vi "Station_2_Home_Data.vi"(8 "Loader Home Data IN":T1={"Approach Velocity\n(In/Sec)"=1.0, "Creep Velocity\n(In/Sec)"=0.5, "Offset (In)"=0.0625, "OffsetVelocity\n(In/Sec)"=0.5, "AccDec\n(In/Sec/Sec)"=1.0, "Position (In)"=0.0} {"Position (In)" min=0.0 max=1.0 format="%.3f"; "AccDec\n(In/Sec/Sec)" min=0.01 max=20.0 format="%.2f"; "OffsetVelocity\n(In/Sec)" min=0.01 max=2.0 format="%.2f"; "Offset (In)" min=-1.0 max=1.0 format="%.3f"; "Creep Velocity\n(In/Sec)" min=0.5 max=1.0 format="%.2f"; "Approach Velocity\n(In/Sec)" min=0.01 max=2.0 format="%.2f"}, 9 "Z Home Data IN":T1={"Approach Velocity\n(In/Sec)"=1.0, "Creep Velocity\n(In/Sec)"=0.5, "Offset (In)"=-0.0625, "OffsetVelocity\n(In/Sec)"=0.5, "AccDec\n(In/Sec/Sec)"=1.0, "Position (In)"=5.75} {"Position (In)" format="%.3f"; "AccDec\n(In/Sec/Sec)" min=0.01 max=20.0 format="%.2f"; "OffsetVelocity\n(In/Sec)" min=0.01 max=2.0 format="%.2f"; "Offset (In)" min=-1.0 format="%.3f"; "Creep Velocity\n(In/Sec)" min=0.5 max=1.0 format="%.2f"; "Approach Velocity\n(In/Sec)" min=0.01 max=2.0 format="%.2f"}, 10 "Y Home Data IN":T1={"Approach Velocity\n(In/Sec)"=1.0, "Creep Velocity\n(In/Sec)"=0.5, "Offset (In)"=-0.0625, "OffsetVelocity\n(In/Sec)"=0.5, "AccDec\n(In/Sec/Sec)"=1.0, "Position (In)"=5.9} {"Position (In)" format="%.3f"; "AccDec\n(In/Sec/Sec)" min=0.01 max=20.0 format="%.2f"; "OffsetVelocity\n(In/Sec)" min=0.01 max=2.0 format="%.2f"; "Offset (In)" min=-1.0 max=1.0 format="%.3f"; "Creep Velocity\n(In/Sec)" min=0.5 max=1.0 format="%.2f"; "Approach Velocity\n(In/Sec)" min=0.01 max=2.0 format="%.2f"}, 11 "X Home Data IN":T2={"Approach Velocity (In/Sec)"=1.0, "Creep Velocity (In/Sec)"=0.5, "Offset (In)"=-0.0625, "OffsetVelocity (In/Sec)"=0.5, "AccDec\n(In/Sec/Sec)"=1.0, "Position (In)"=22.525} {"Position (In)" format="%.3f"; "AccDec\n(In/Sec/Sec)" min=0.01 max=20.0 format="%.2f"; "OffsetVelocity (In/Sec)" min=0.01 max=2.0 format="%.2f"; "Offset (In)" min=-1.0 max=1.0 format="%.3f"; "Creep Velocity (In/Sec)" min=0.5 max=1.0 format="%.2f"; "Approach Velocity (In/Sec)" min=0.01 max=2.0 format="%.2f"}) -> (0 "Loader Home Data OUT":T1={"Approach Velocity\n(In/Sec)"=nan, "Creep Velocity\n(In/Sec)"=nan, "Offset (In)"=nan, "OffsetVelocity\n(In/Sec)"=nan, "AccDec\n(In/Sec/Sec)"=nan, "Position (In)"=nan} {"Position (In)" min=0.0 max=1.0 format="%.3f"; "AccDec\n(In/Sec/Sec)" min=0.01 max=20.0 format="%.2f"; "OffsetVelocity\n(In/Sec)" min=0.01 max=2.0 format="%.2f"; "Offset (In)" min=-1.0 max=1.0 format="%.3f"; "Creep Velocity\n(In/Sec)" min=0.5 max=1.0 format="%.2f"; "Approach Velocity\n(In/Sec)" min=0.01 max=2.0 format="%.2f"}, 1 "Z Home Data OUT":T1={"Approach Velocity\n(In/Sec)"=nan, "Creep Velocity\n(In/Sec)"=nan, "Offset (In)"=nan, "OffsetVelocity\n(In/Sec)"=nan, "AccDec\n(In/Sec/Sec)"=nan, "Position (In)"=nan} {"Position (In)" format="%.3f"; "AccDec\n(In/Sec/Sec)" min=0.01 max=20.0 format="%.2f"; "OffsetVelocity\n(In/Sec)" min=0.01 max=2.0 format="%.2f"; "Offset (In)" min=-1.0 format="%.3f"; "Creep Velocity\n(In/Sec)" min=0.5 max=1.0 format="%.2f"; "Approach Velocity\n(In/Sec)" min=0.01 max=2.0 format="%.2f"}, 2 "Y Home Data OUT":T1={"Approach Velocity\n(In/Sec)"=nan, "Creep Velocity\n(In/Sec)"=nan, "Offset (In)"=nan, "OffsetVelocity\n(In/Sec)"=nan, "AccDec\n(In/Sec/Sec)"=nan, "Position (In)"=nan} {"Position (In)" format="%.3f"; "AccDec\n(In/Sec/Sec)" min=0.01 max=20.0 format="%.2f"; "OffsetVelocity\n(In/Sec)" min=0.01 max=2.0 format="%.2f"; "Offset (In)" min=-1.0 max=1.0 format="%.3f"; "Creep Velocity\n(In/Sec)" min=0.5 max=1.0 format="%.2f"; "Approach Velocity\n(In/Sec)" min=0.01 max=2.0 format="%.2f"}, 3 "X Home Data OUT":T2={"Approach Velocity (In/Sec)"=nan, "Creep Velocity (In/Sec)"=nan, "Offset (In)"=nan, "OffsetVelocity (In/Sec)"=nan, "AccDec\n(In/Sec/Sec)"=nan, "Position (In)"=nan} {"Position (In)" format="%.3f"; "AccDec\n(In/Sec/Sec)" min=0.01 max=20.0 format="%.2f"; "OffsetVelocity (In/Sec)" min=0.01 max=2.0 format="%.2f"; "Offset (In)" min=-1.0 max=1.0 format="%.3f"; "Creep Velocity (In/Sec)" min=0.5 max=1.0 format="%.2f"; "Approach Velocity (In/Sec)" min=0.01 max=2.0 format="%.2f"})   [LabVIEW 2010]
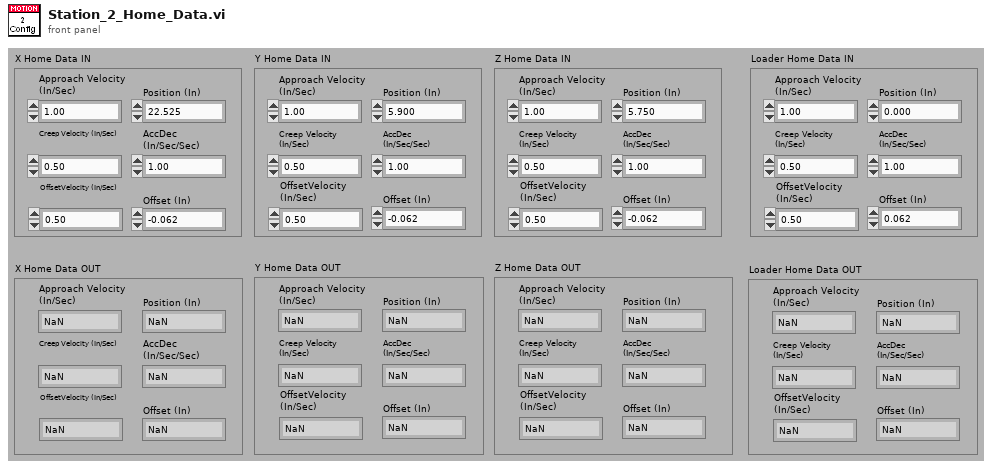
[diagram p1: front panel]
types:
  T1 = cluster{"Approach Velocity\n(In/Sec)":dbl, "Creep Velocity\n(In/Sec)":dbl, "Offset (In)":dbl, "OffsetVelocity\n(In/Sec)":dbl, "AccDec\n(In/Sec/Sec)":dbl, "Position (In)":dbl}
  T2 = cluster{"Approach Velocity (In/Sec)":dbl, "Creep Velocity (In/Sec)":dbl, "Offset (In)":dbl, "OffsetVelocity (In/Sec)":dbl, "AccDec\n(In/Sec/Sec)":dbl, "Position (In)":dbl}
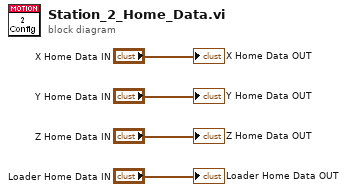
[diagram p0: block diagram]
diagram:
  "X Home Data OUT" <- "X Home Data IN"
  "Y Home Data OUT" <- "Y Home Data IN"
  "Z Home Data OUT" <- "Z Home Data IN"
  "Loader Home Data OUT" <- "Loader Home Data IN"
